vi "System State Broadcast Helper Loop Timeout.vi"() -> (3 "timeout":i32)   [LabVIEW 2024, in "Hardware Controller.lvlib"]
uses:
  Hardware Controller.lvlib
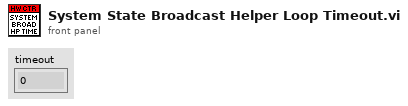
[diagram p1: front panel]
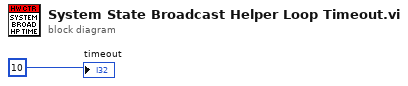
[diagram p0: block diagram]
diagram:
  "timeout" <- 10
